vi "ChassisSystemSet4Deadbands.vi"(0 "Inputs":dbl[](array[numeric]), 1 "Deadband":dbl) -> (2 "Output 1":dbl, 3 "Output 2":dbl, 4 "Output 3":dbl, 5 "Output 4":dbl)   [LabVIEW 2014]
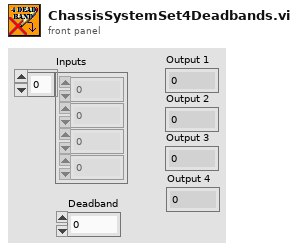
[diagram p1: front panel]
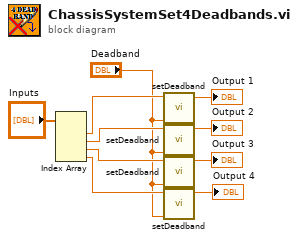
[diagram p0: block diagram]
diagram:
  n1 = Index Array(array="Inputs") -> (element #1=w7:dbl, element #2=w6:dbl, element #3=w9:dbl, element #4=w8:dbl)  [unwired: 4 in]
  n2 = call "setDeadband.vi"("Deadband"="Deadband", "Joystick Axis Value"=w7) -> ("Output Motor Value"=→"Output 1":dbl)  [unwired: 9 in]
  n3 = call "setDeadband.vi"("Deadband"="Deadband", "Joystick Axis Value"=w6) -> ("Output Motor Value"=→"Output 2":dbl)  [unwired: 9 in]
  n4 = call "setDeadband.vi"("Deadband"="Deadband", "Joystick Axis Value"=w9) -> ("Output Motor Value"=→"Output 3":dbl)  [unwired: 9 in]
  n5 = call "setDeadband.vi"("Deadband"="Deadband", "Joystick Axis Value"=w8) -> ("Output Motor Value"=→"Output 4":dbl)  [unwired: 9 in]
